vi "Flat_Sequence_Str.vi"() -> ()   [LabVIEW 2019]
panel:
  out "Indicator":i32
  in  "stop":bool
  out "Add Array":dbl[](array[numeric])
  in  "Array 3":dbl[](array[numeric])
  in  "Array 2":dbl[](array[numeric])
  out "size(s)":i32
  in  "Array":dbl[](array[numeric])
  # "Array Size"
  # "Array Addition"
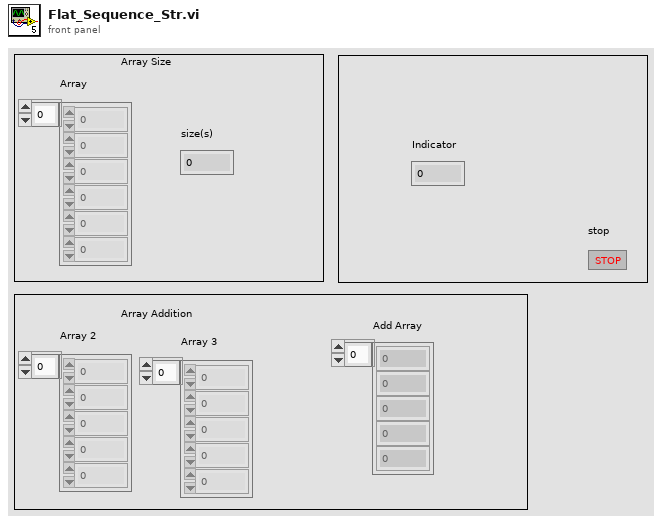
[diagram p1: front panel]
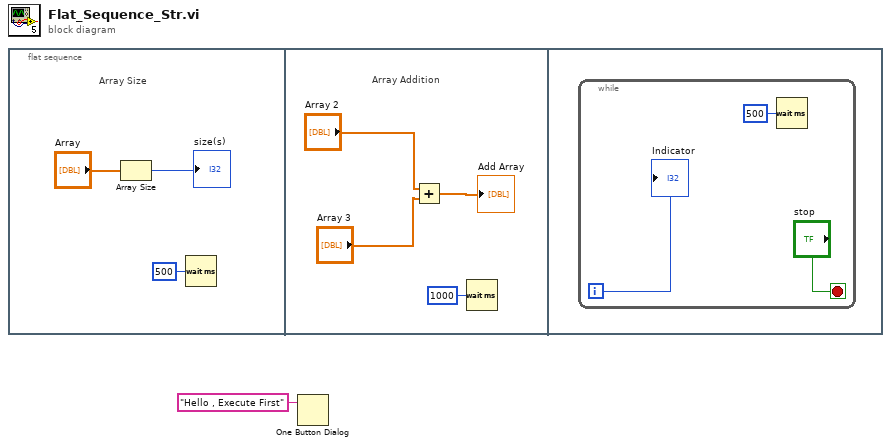
[diagram p0: block diagram]
diagram:
  n1 = flat-sequence {
    frame #0 {
      # "Array Size"
      n2 = Array Size(array="Array") -> (size(s)=→"size(s)":i32)
      n3 = Wait (ms)(milliseconds to wait=u32 500) -> ()  [unwired: 1 out]
    }
    frame #1 {
      # "Array Addition"
      n4 = Add(x="Array 2", y="Array 3") -> (x+y=→"Add Array":dbl[])
      n5 = Wait (ms)(milliseconds to wait=u32 1000) -> ()  [unwired: 1 out]
    }
    frame #2 {
      n6 = while {
        i -> [w10]
        stop <- "stop" stop-if-true
        n7 = Wait (ms)(milliseconds to wait=u32 500) -> ()  [unwired: 1 out]
        "Indicator" <- w10
      }
    }
  }
  n8 = One Button Dialog(message="Hello , Execute First") -> ()  [unwired: 1 in, 1 out]
